vi "Go To Starting Command.vi"(8 "error in (no error)":errorcluster, 11 "Command States in":refnum<class "Command States.lvclass">) -> (0 "error out":errorcluster, 3 "State out":refnum<class "State Actor.lvclass">)   [LabVIEW 2013, in "Command Actor.lvlib" / "Command States.lvclass"]
uses:
  Command States.lvclass
  <vilib>/ni/Actors/State Actor/State Actor/State Actor.lvclass
  Starting Command/Starting Command.lvclass
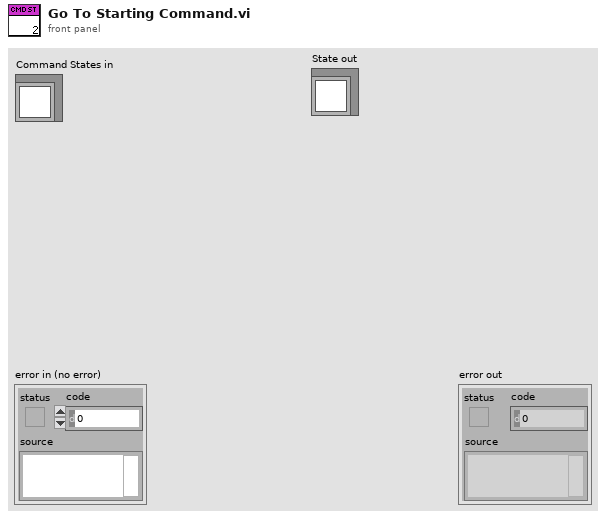
[diagram p1: front panel]
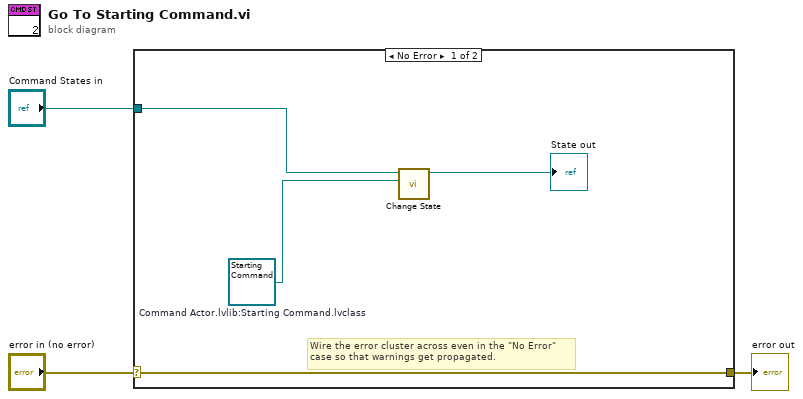
[diagram p0: block diagram]
diagram:
  n1 = case shown="No Error" "error in (no error)" {
    selector: "error in (no error)" -> [w7 w8]
    tunnel: [w7 w8] -> w2
    tunnel: "Command States in" -> [w6 _]
    frame No Error {
      w5 = refnum<class "Starting Command.lvclass"> refnum  # Command Actor.lvlib:Starting Command.lvclass
      # "Wire the error cluster across even in the \"No Error\"\ncase so that warnings get propagated."
      n2 = call <vilib>:"Change State.vi"("New State in"=w5, "State in"=w6) -> ("State out"=→"State out":refnum<class "State Actor.lvclass">)  [unwired: 8 in, 1 out]
    }
    frame Error {
    }
  }
  "error out" <- w2
